vi "lectura img.vi"() -> ()   [LabVIEW 2020]
panel:
  in  "Slide 2":u8(slide) scale=0.0..255.0
  in  "Slide":u8(slide) scale=0.0..255.0
  in  "Path":path
  out "new picture":picture
  # "Ceballos Conde Emanuel"
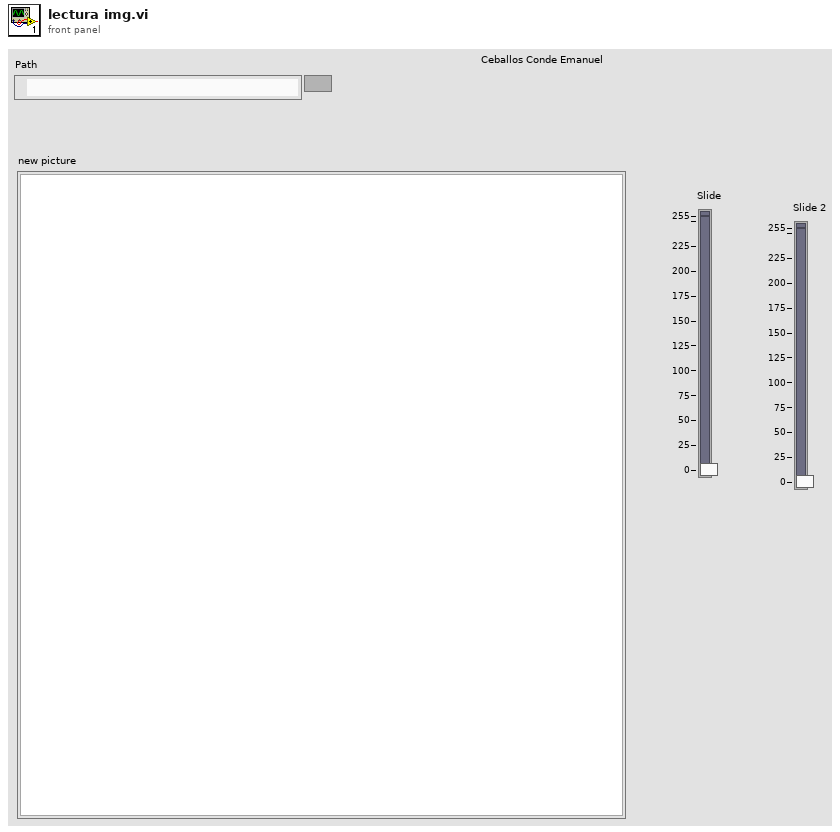
[diagram p1: front panel]
types:
  T1 = typedef "imagedata.ctl" = cluster{"image type":i32, "image depth":i32, "image":u8[], "mask":u8[], "colors":u32[], "Rectangle":cluster{"left":i16, "top":i16, "right":i16, "bottom":i16}}
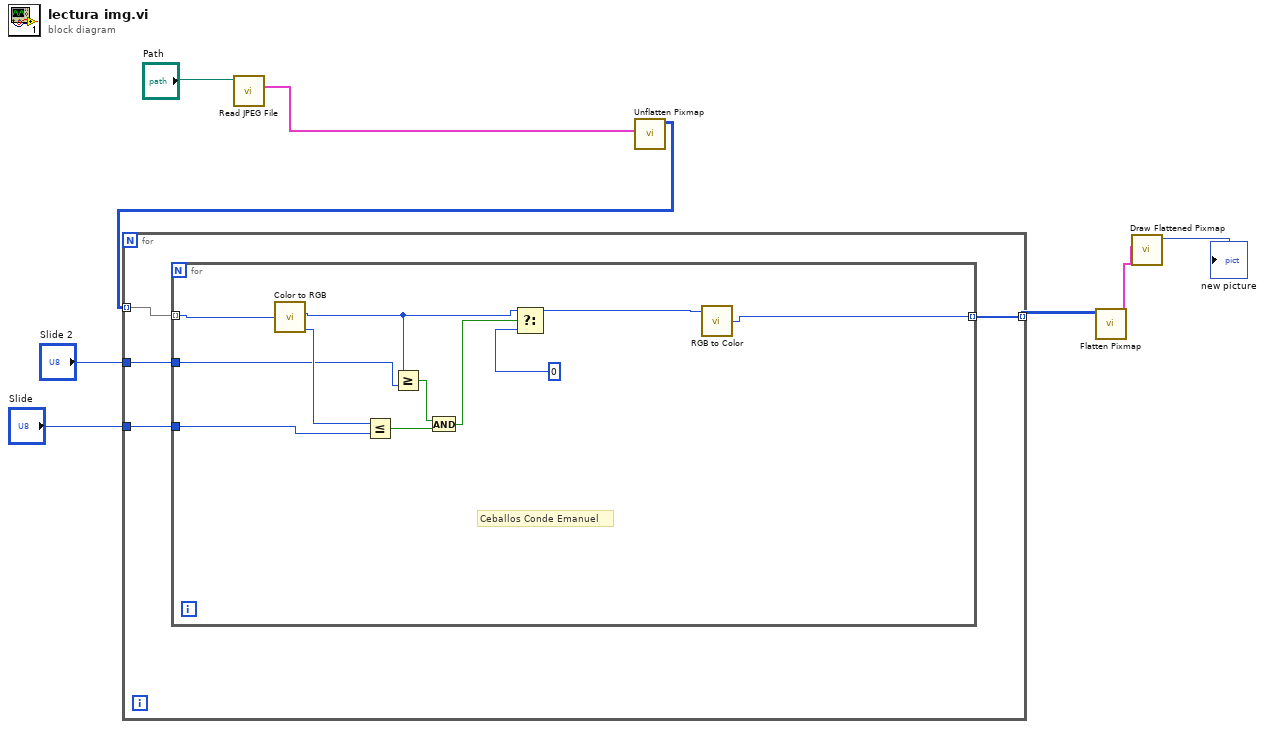
[diagram p0: block diagram]
diagram:
  n1 = call <vilib>:"Read JPEG File.vi"("path to JPEG file"="Path") -> ("image data"=w7:T1)  [unwired: 8 in, 2 out]
  n2 = call <vilib>:"Unflatten Pixmap.vi"("image data"=w7) -> ("24-bit pixmap"=w6:u32[][])  [unwired: 4 in, 6 out]
  n3 = for {
    tunnel: w6 -> [w12] mode=indexing
    tunnel: [w11] -> w4 mode=indexing
    tunnel: "Slide" -> [w10]
    tunnel: "Slide 2" -> [w9]
    n4 = for {
      tunnel: w12 -> [w23] mode=indexing
      tunnel: [w22] -> w11 mode=indexing
      tunnel: w10 -> [w21]
      tunnel: w9 -> [w17]
      # "Ceballos Conde Emanuel"
      n5 = call <vilib>:"Color to RGB.vi"("Color"=w23) -> ("R"=w13:u8, "B"=w18:u8)  [unwired: 2 out]
      n6 = Less Or Equal?(x=w18, y=w21) -> (x <= y?=w15:bool)
      n7 = Greater Or Equal?(x=w13, y=w17) -> (x >= y?=w16:bool)
      n8 = And(x=w16, y=w15) -> (x .and. y?=w14:bool)
      n9 = Select(t=w13, s=w14, f=u8 0 ("B")) -> (s? t:f=w19:u8)
      n10 = call <vilib>:"RGB to Color.vi"("R"=w19) -> ("Color"=w22:u32)  [unwired: 2 in]
    }
  }
  n11 = call <vilib>:"Flatten Pixmap.vi"("24-bit pixmap"=w4) -> ("image data"=w5:T1)  [unwired: 10 in]
  n12 = call <vilib>:"Draw Flattened Pixmap.vi"("image data"=w5) -> ("new picture"=→"new picture":picture)  [unwired: 8 in]
